vi "Tag Write to File.vi"(8 "error in (no error)":errorcluster, 9 "Pending data in":refnum<data-value>[](array[refnum]), 10 "refnum in":refnum<file>, 11 "IFD_Tag in":refnum<class "IFD_Tag.lvclass">) -> (0 "error out":errorcluster, 1 "Pending data out":refnum<data-value>[](array[refnum]), 2 "refnum out":refnum<file>)   [LabVIEW 2016, in "IFD_Tag.lvclass"]
uses:
  IFD_Tag.lvclass
  Offset Content.ctl
  IFD_Tag.lvclass/IFD_Tag.ctl
panel:
  out "data string 4":string
  out "data string 3":string
  out "concatenated string":string
  out "data string 2":string
  out "data string":string
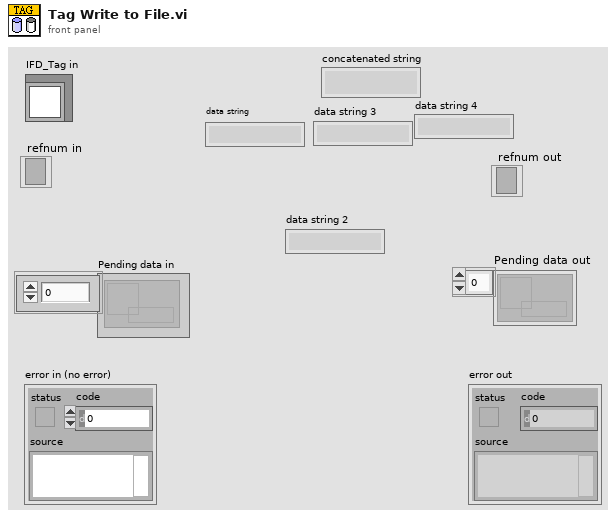
[diagram p1: front panel]
types:
  T1 = enum16{"big-endian, network order", "native, host order", "little-endian"}
  T2 = typedef "Offset Content.ctl" = cluster{"Pointer Byte Offset":u32, "Content":string}
  T3 = enum16{"Undefined(DO NOT USE)", "U8", "ASCII", "U16", "U32", "RATIONAL", "I8", "Undefined 8 bit", "I16", "I32", "SRATIONAL", "SGL", "DBL"}
  T4 = cluster{"Tag ID":u16, "Data Type":enum16{"Undefined(DO NOT USE)", "U8", "ASCII", "U16", "U32", "RATIONAL", "I8", "Undefined 8 bit", "I16", "I32", "SRATIONAL", "SGL", "DBL"}, "Data Count":u32}
  T5 = cluster{"Tag ID":u16, "Data Type":enum16{"Undefined(DO NOT USE)", "U8", "ASCII", "U16", "U32", "RATIONAL", "I8", "Undefined 8 bit", "I16", "I32", "SRATIONAL", "SGL", "DBL"}, "Data Count":u32, u32}
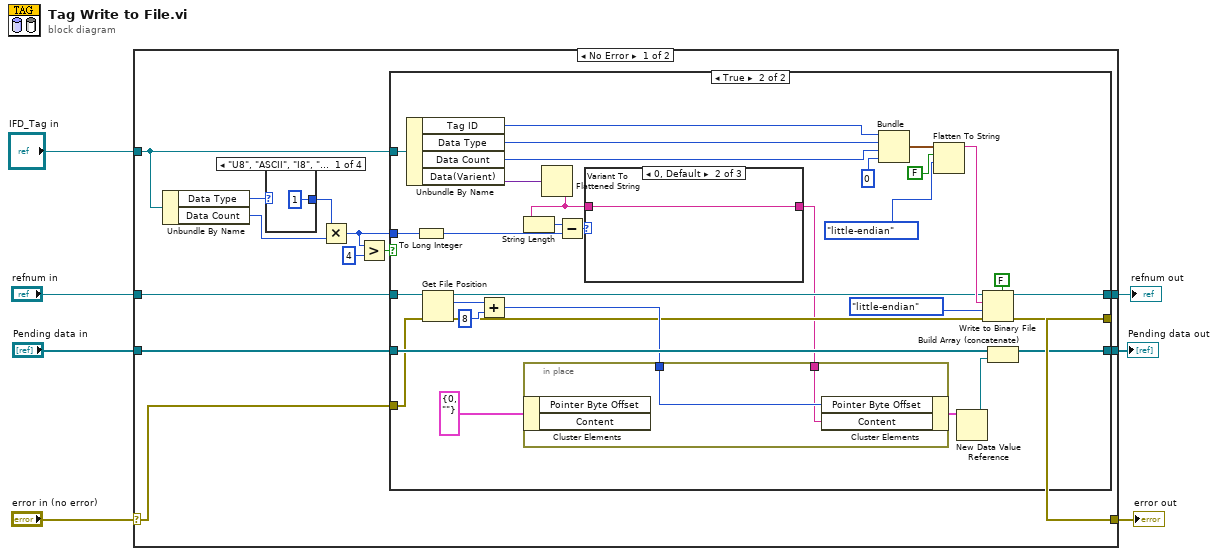
[diagram p0: block diagram]
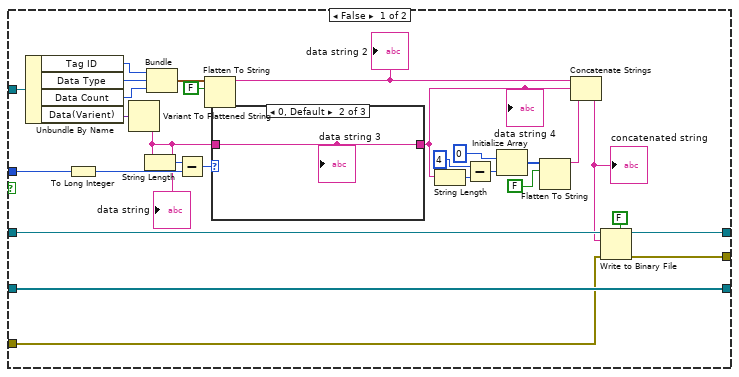
[diagram p2: hidden frame]
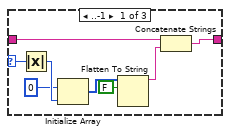
[diagram p3: hidden frame]
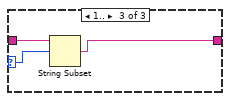
[diagram p4: hidden frame]
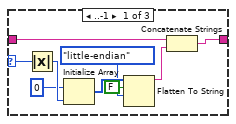
[diagram p5: hidden frame]
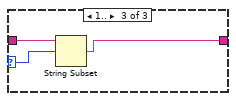
[diagram p6: hidden frame]
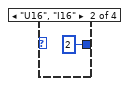
[diagram p7: hidden frame]
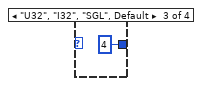
[diagram p8: hidden frame]
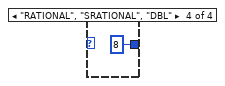
[diagram p9: hidden frame]
diagram:
  n1 = case shown="No Error" "error in (no error)" {
    selector: "error in (no error)" -> [w11 w114]
    tunnel: [w9 w114] -> w6
    tunnel: "IFD_Tag in" -> [w15 _]
    tunnel: "Pending data in" -> [w13 w112]
    tunnel: "refnum in" -> [w14 w113]
    tunnel: [w12 w112] -> w2
    tunnel: [w10 w113] -> w1
    frame No Error {
      n2 = Unbundle By Name(w15) -> ("Data Type"=w20:T3, "Data Count"=w17:u32)
      n3 = case shown="\"U8\", \"ASCII\", \"I8\", \"Undefined 8 bit\"" w20 {
        tunnel: [u32 1 u32 2 u32 4 u32 8] -> w19
        frame "U8", "ASCII", "I8", "Undefined 8 bit" {
        }
        frame "U16", "I16" {
        }
        frame "U32", "I32", "SGL", Default {
        }
        frame "RATIONAL", "SRATIONAL", "DBL" {
        }
      }
      n4 = Multiply(x=w19, y=w17) -> (x*y=w8:u32)
      n5 = Greater?(x=w8, y=u32 4) -> (0:w16:bool)
      n6 = case shown="True" w16 {
        tunnel: w15 -> [w48 w92]
        tunnel: w14 -> [w47 w82]
        tunnel: w13 -> [w45 w78]
        tunnel: [w45 w76] -> w12
        tunnel: w11 -> [w35 w72]
        tunnel: [w36 w85] -> w10
        tunnel: [w34 w70] -> w9
        tunnel: w8 -> [w30 w68]
        frame False {
          n7 = Unbundle By Name(w48) -> ("Tag ID"=w43:u16, "Data Type"=w42:T3, "Data Count"=w41:u32, "Data(Varient)"=w44:variant)
          n8 = To Long Integer(number=w30) -> (32bit integer=w32:i32)
          n9 = Variant To Flattened String(Variant=w44) -> (data string=w29:string)  [unwired: 1 out]
          "data string" <- w29
          n10 = String Length(string=w29) -> (length=w31:i32)
          n11 = Bundle("Tag ID"=w43, "Data Type"=w42, "Data Count"=w41) -> (w40:T4)  [unwired: 1 in]
          n12 = Subtract(x=w31, y=w32) -> (x-y=w33:i32)
          n13 = Flatten To String(anything=w40, prepend array or string size? (T)=FALSE) -> (data string=w38:string)  [unwired: 2 in, 2 out]
          "data string 2" <- w38
          n14 = case shown="0, Default" w33 {
            selector: w33 -> [w56 _ w59]
            tunnel: w29 -> [w51 w57 w60]
            tunnel: [w49 w57 w58] -> w26
            frame ..-1 {
              n15 = Absolute Value(x=w56) -> (abs(x)=w55:i32)
              n16 = Initialize Array(u8 0, w55) -> (w53:u8[])
              n17 = Flatten To String(anything=w53, prepend array or string size? (T)=FALSE) -> (data string=w50:string)  [unwired: 2 in, 2 out]
              n18 = Concatenate Strings(w51, w50) -> (w49:string)
            }
            frame 0, Default {
              "data string 3" <- w57
            }
            frame 1.. {
              n19 = String Subset(string=w60, offset (0)=w59) -> (substring=w58:string)  [unwired: 1 in]
            }
          }
          "data string 4" <- w26
          n20 = String Length(string=w26) -> (length=w28:i32)
          n21 = Subtract(x=4 ("y"), y=w28) -> (x-y=w25:i32)
          n22 = Initialize Array(u8 0, w25) -> (w23:u8[])
          n23 = Flatten To String(anything=w23, prepend array or string size? (T)=FALSE) -> (data string=w22:string)  [unwired: 2 in, 2 out]
          n24 = Concatenate Strings(w38, w26, w22) -> (w37:string)
          "concatenated string" <- w37
          n25 = Write to Binary File(file (use dialog)=w47, data=w37, error in=w35, 5:FALSE) -> (refnum out=w36:refnum<file>, error out=w34:errorcluster)  [unwired: 2 in, 1 out]
        }
        frame True {
          n26 = Unbundle By Name(w92) -> ("Tag ID"=w90:u16, "Data Type"=w89:T3, "Data Count"=w88:u32, "Data(Varient)"=w69:variant)
          n27 = To Long Integer(number=w68) -> (32bit integer=w66:i32)
          n28 = Get File Position(4:w72, 7:w82) -> (0:w71:errorcluster, 2:w80:i64, 3:w81:refnum<file>)
          n29 = Add(x=w80, y=i64 8) -> (x+y=w73:i64)
          n30 = Variant To Flattened String(Variant=w69) -> (data string=w64:string)  [unwired: 1 out]
          n31 = String Length(string=w64) -> (length=w67:i32)
          n32 = Subtract(x=w67, y=w66) -> (x-y=w65:i32)
          n33 = case shown="0, Default" w65 {
            selector: w65 -> [w101 _ w104]
            tunnel: w64 -> [w96 w102 w105]
            tunnel: [w94 w102 w103] -> w63
            frame ..-1 {
              n34 = Absolute Value(x=w101) -> (abs(x)=w100:i32)
              n35 = Initialize Array(u8 0, w100) -> (w98:u8[])
              n36 = Flatten To String(anything=w98, prepend array or string size? (T)=FALSE, byte order (0:big-endian, network order)=T1."little-endian") -> (data string=w95:string)  [unwired: 1 in, 2 out]
              n37 = Concatenate Strings(w96, w95) -> (w94:string)
            }
            frame 0, Default {
            }
            frame 1.. {
              n38 = String Subset(string=w105, offset (0)=w104) -> (substring=w103:string)  [unwired: 1 in]
            }
          }
          n39 = in-place {
            in-place-border: w73 -> [w107]
            in-place-border: w63 -> [w106]
            n40 = in-place-cluster #1(T2 {"Pointer Byte Offset"=0, "Content"=""} ("Offset Content")) -> ()  [unwired: 2 out]
            n41 = in-place-cluster #1("Pointer Byte Offset"=w107, "Content"=w106) -> (w74:T2)
          }
          n42 = Bundle("Tag ID"=w90, "Data Type"=w89, "Data Count"=w88, u32 0) -> (w87:T5)  [unwired: 1 in]
          n43 = Flatten To String(anything=w87, prepend array or string size? (T)=FALSE, byte order (0:big-endian, network order)=T1."little-endian") -> (data string=w83:string)  [unwired: 1 in, 2 out]
          n44 = New Data Value Reference(data value=w74) -> (data value reference=w77:refnum<data-value>)  [unwired: 1 in, 1 out]
          n45 = Write to Binary File(file (use dialog)=w81, data=w83, error in=w71, 5:FALSE, 9:T1."little-endian" ("byte order (0:big-endian, network order)")) -> (refnum out=w85:refnum<file>, error out=w70:errorcluster)  [unwired: 1 in, 1 out]
          n46 = Build Array (concatenate)(w78, w77) -> (w76:refnum<data-value>[])
        }
      }
    }
    frame Error {
    }
  }
  "error out" <- w6
  "Pending data out" <- w2
  "refnum out" <- w1
